vi "Read Data.vi"(1 "Channel Number":i32, 2 "GPIB Address":string, 3 "Number of Datapoints":i32) -> (0 "Data":i32[](array[numeric]))   [LabVIEW 2015, in "SR400.lvlib"]
uses:
  SR400.lvlib
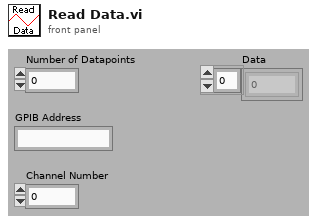
[diagram p1: front panel]
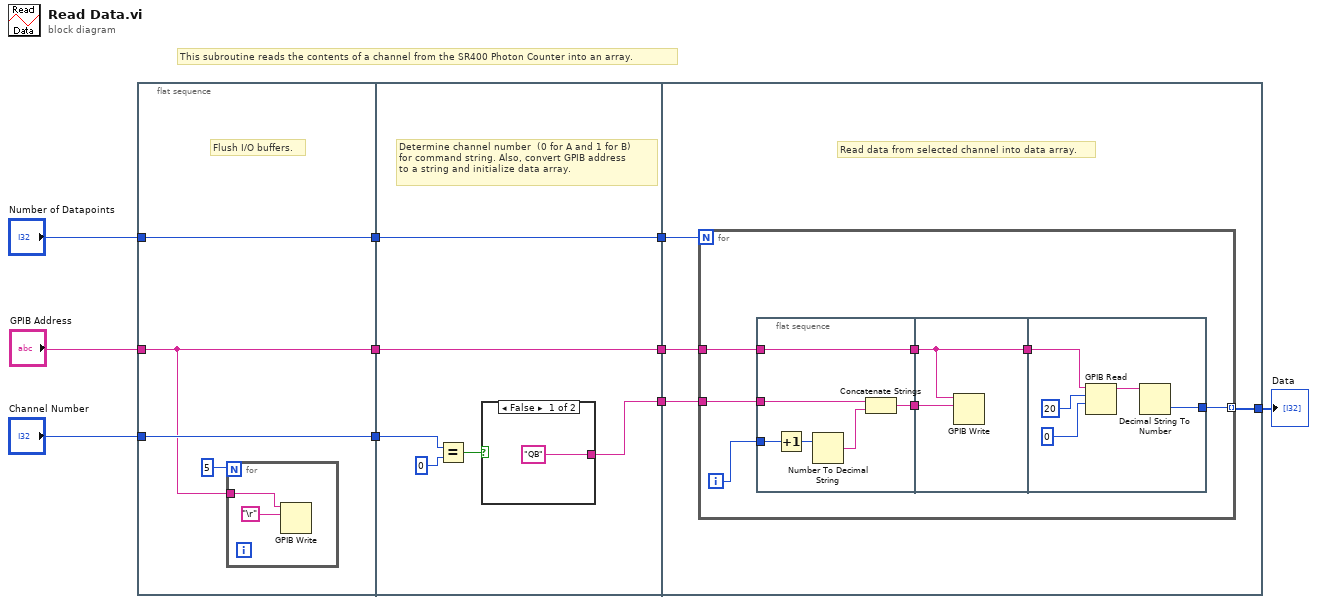
[diagram p0: block diagram]
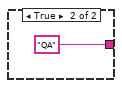
[diagram p2: hidden frame]
diagram:
  # "This subroutine reads the contents of a channel from the SR400 Photon Counter into an array."
  n1 = flat-sequence {
    tunnel: "GPIB Address" -> [w11]
    tunnel: "Number of Datapoints" -> [w13]
    tunnel: "Channel Number" -> [w14]
    tunnel: [w14] -> w3
    tunnel: [w13] -> w2
    tunnel: [w11] -> w1
    tunnel: [w19] -> w7
    tunnel: [w18] -> w6
    tunnel: [w17] -> w5
    tunnel: w3 -> [w20]
    tunnel: w2 -> [w17]
    tunnel: w1 -> [w18]
    tunnel: w7 -> [w28]
    tunnel: w6 -> [w27]
    tunnel: w5 -> [w26]
    tunnel: [w25] -> w4
    frame #0 {
      # "Flush I/O buffers."
      n2 = for {
        N: 5 -> [_]
        tunnel: w11 -> [w16]
        n3 = GPIB Write(0:w16, 1:"\r") -> ()  [unwired: 3 in, 2 out]
      }
    }
    frame #1 {
      # "Determine channel number  (0 for A and 1 for B) \nfor command string. Also, convert GPIB address\nto a string and initialize data array."
      n4 = Equal?(x=w20, y=0) -> (x = y?=w22:bool)
      n5 = case shown="False" w22 {
        tunnel: ["QB" "QA"] -> w19
        frame False {
        }
        frame True {
        }
      }
    }
    frame #2 {
      # "Read data from selected channel into data array."
      n6 = for {
        N: w26 -> [_]
        tunnel: w28 -> [w34]
        tunnel: w27 -> [w32]
        tunnel: [w30] -> w25 mode=indexing
        i -> [w35]
        n7 = flat-sequence {
          tunnel: w35 -> [w39]
          tunnel: w34 -> [w38]
          tunnel: [w37] -> w33
          tunnel: w32 -> [w36]
          tunnel: [w36] -> w31
          tunnel: w33 -> [w43]
          tunnel: w31 -> [w42]
          tunnel: [w42] -> w29
          tunnel: [w45] -> w30
          tunnel: w29 -> [w44]
          frame #0 {
            n8 = Increment(x=w39) -> (x+1=w40:i32)
            n9 = Number To Decimal String(number=w40) -> (decimal integer string=w41:string)  [unwired: 1 in]
            n10 = Concatenate Strings(w38, w41) -> (w37:string)
          }
          frame #1 {
            n11 = GPIB Write(0:w42, 1:w43) -> ()  [unwired: 3 in, 2 out]
          }
          frame #2 {
            n12 = GPIB Read(0:w44, 1:20, 2:0) -> (5:w48:string)  [unwired: 2 in, 2 out]
            n13 = Decimal String To Number(string=w48) -> (number=w45:i32)  [unwired: 2 in, 1 out]
          }
        }
      }
    }
  }
  "Data" <- w4
